vi "1 to 3 Down_movement_v11.vi"(1 "Input pixmap":u8[][](array[numeric]), 2 "start Column":i32) -> (3 "Total point":i32, 4 "moveLog(Row, Col.)":i32[][](array[numeric]), 5 "To:finish Col.":i32, 6 "TapN":dbl)   [LabVIEW 2016]
panel:
  out "i":i32
  out "1forward":u8[](array[numeric])
  out "2forward":u8[](array[numeric])
  out "RupPoint":dbl[](array[numeric]) format="%_3f"
  out "pointLog":u8[](array[numeric])
  out "min. root p.":u8
  out "3×3 point array":u8[][][](array[numeric])
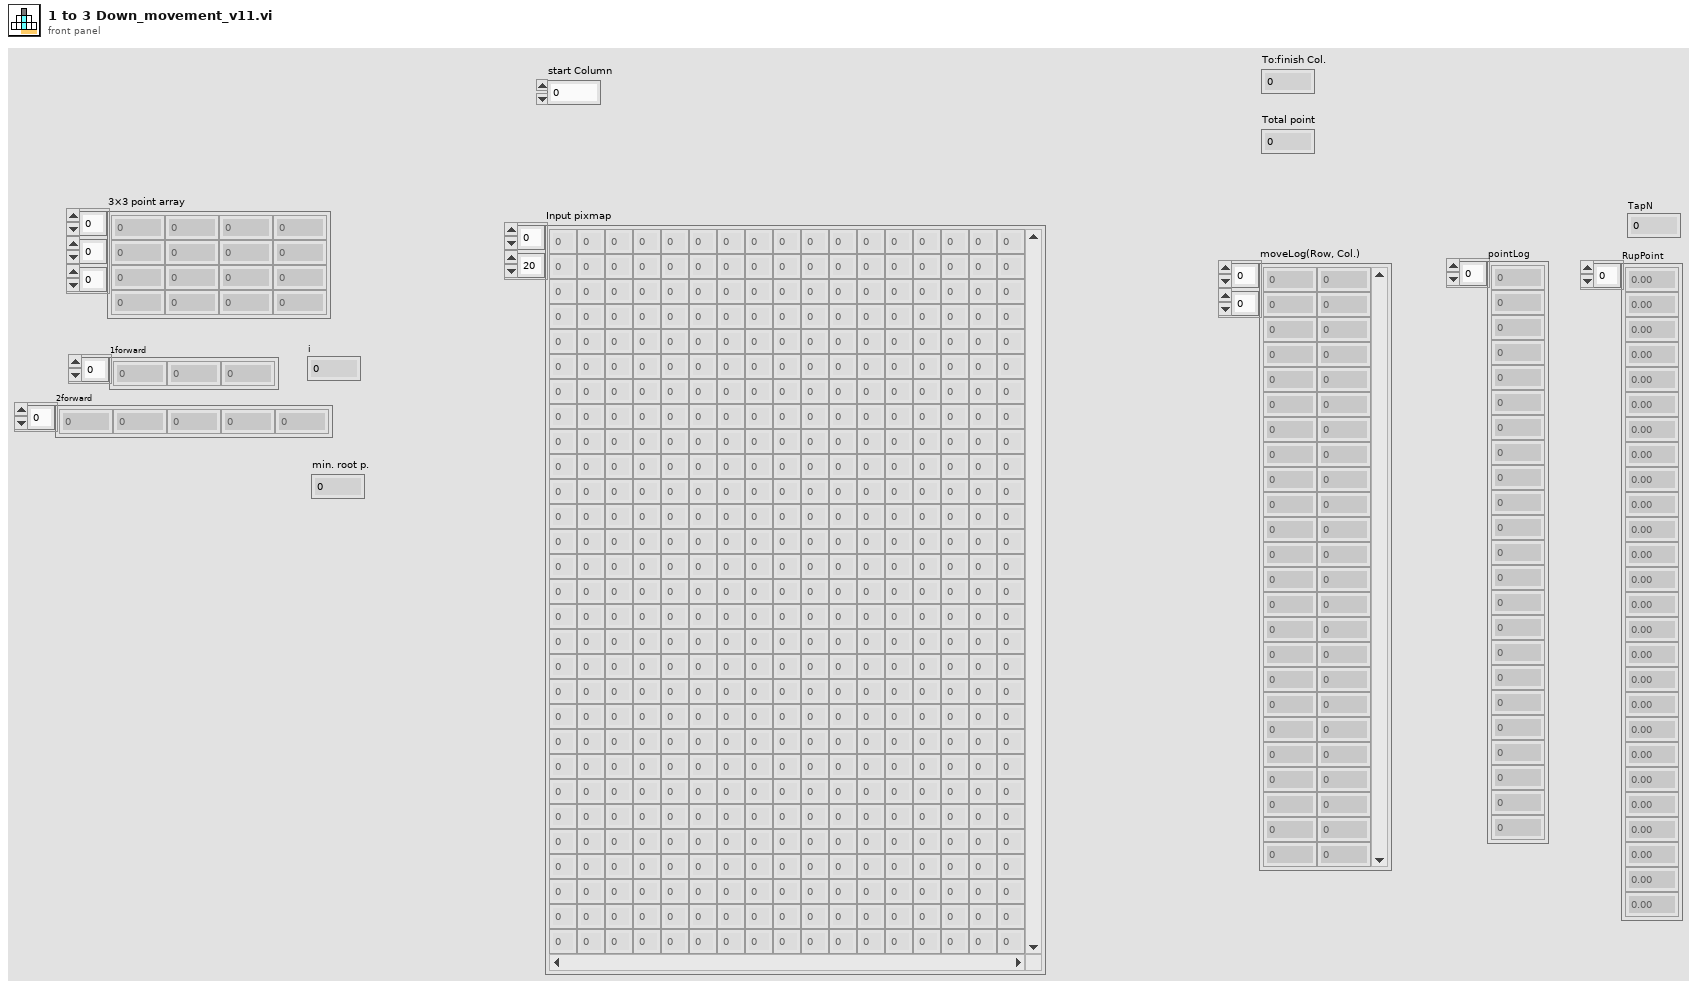
[diagram p1: front panel]
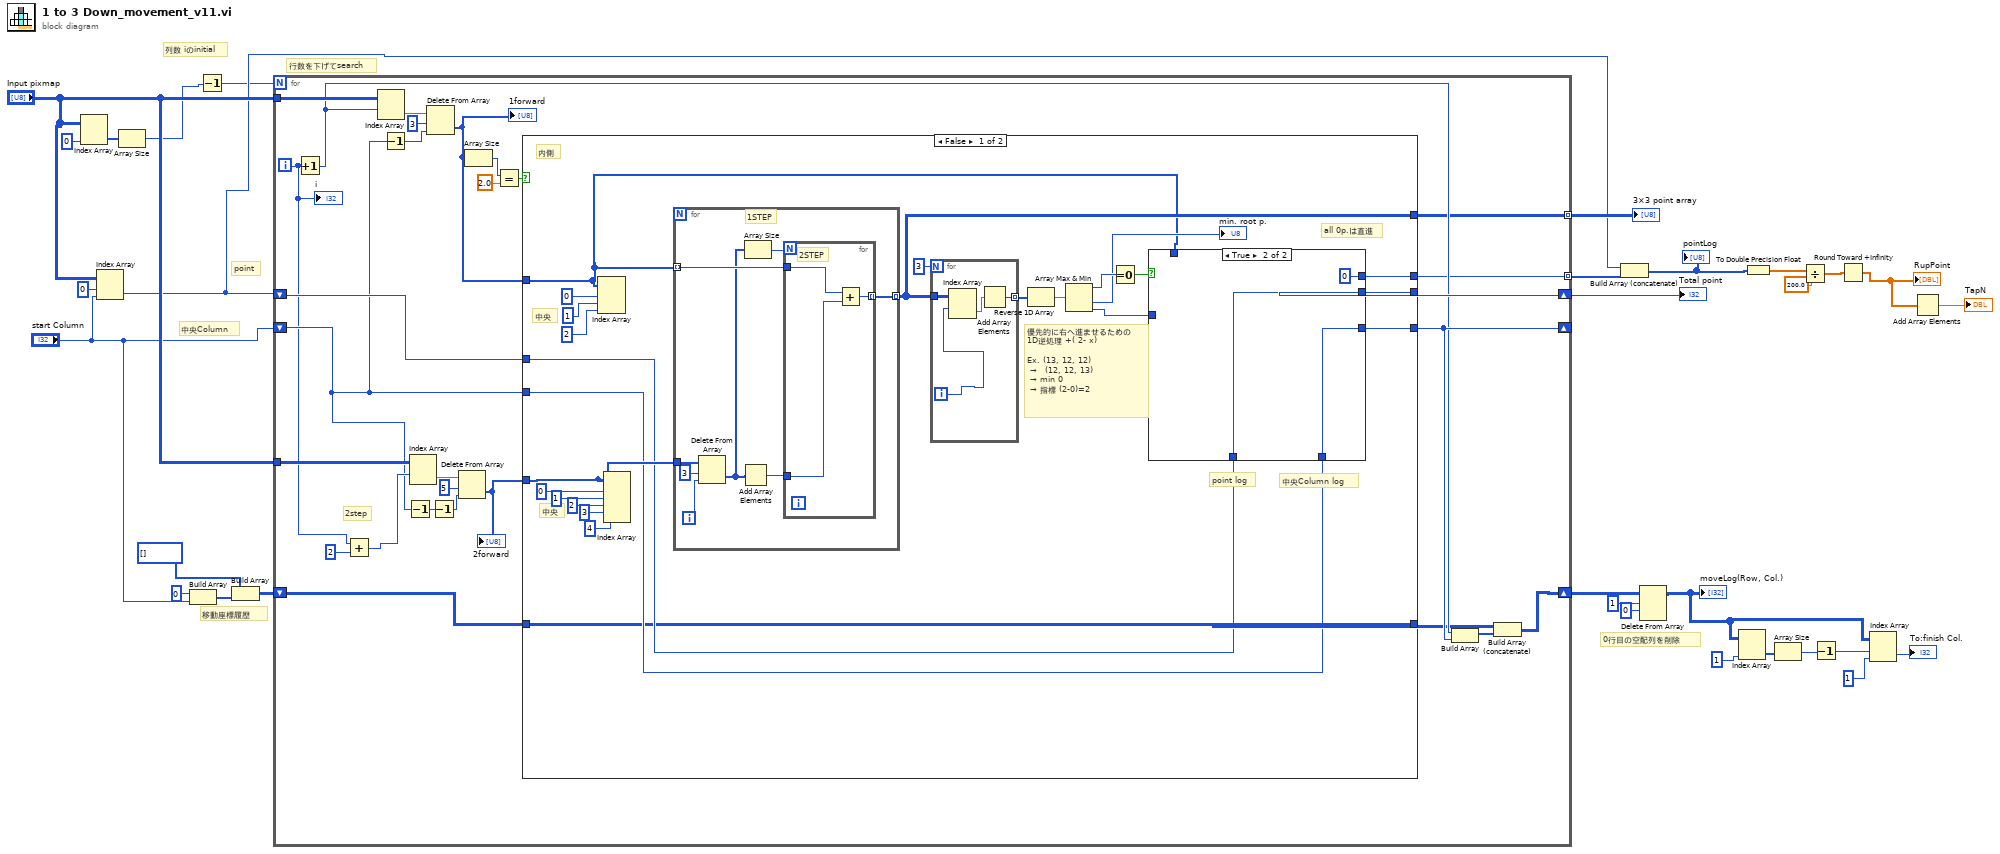
[diagram p0: block diagram]
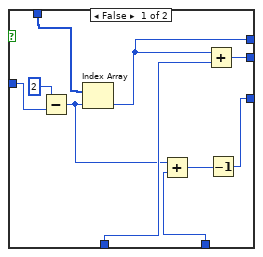
[diagram p2: hidden frame]
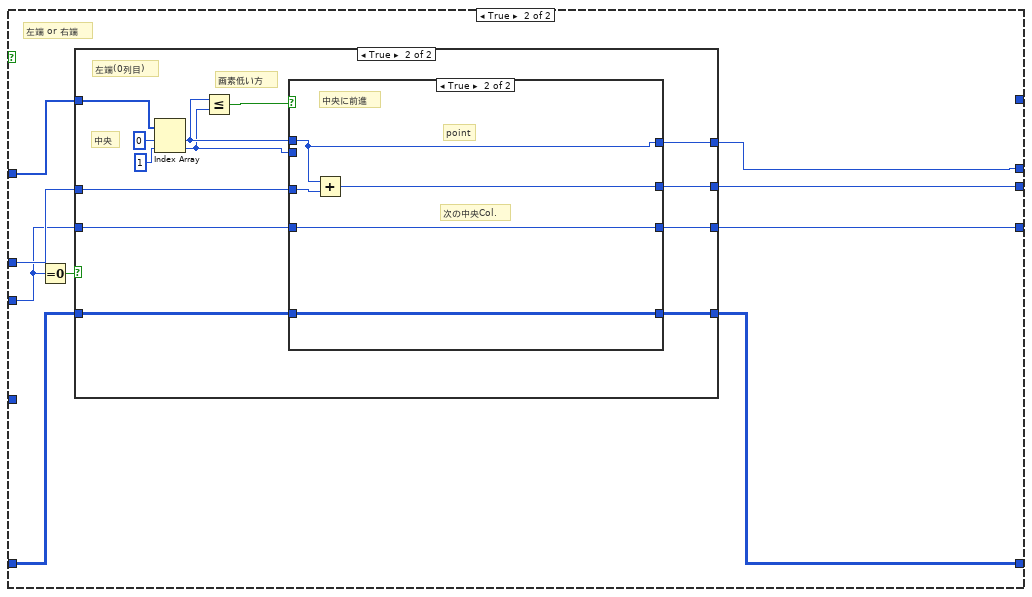
[diagram p3: hidden frame]
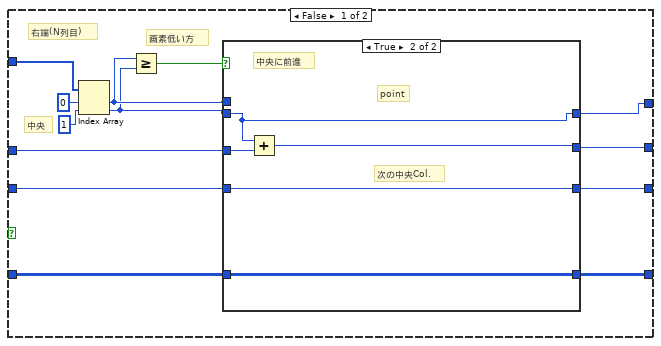
[diagram p4: hidden frame]
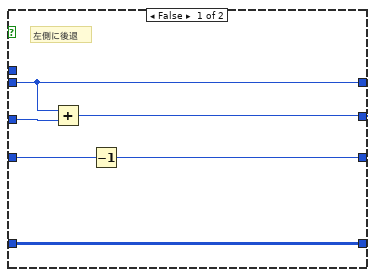
[diagram p5: hidden frame]
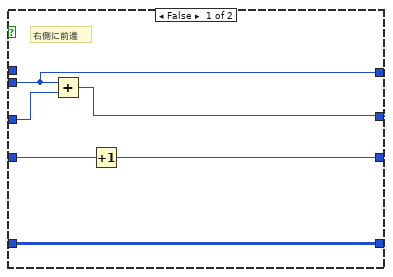
[diagram p6: hidden frame]
diagram:
  # "0行目の空配列を削除"
  # "移動座標履歴"
  # "中央Column"
  # "point"
  # "行数を下げてsearch"
  # "列数 iのinitial"
  n1 = Index Array(array="Input pixmap", index (col)=0 ("無効な指標 （列）")) -> (element=w29:u8[])  [unwired: 1 in]
  n2 = Index Array(array="Input pixmap", index (row)=0 ("指標 （行）"), index (col)="start Column") -> (element=w10:u8)
  n3 = Array Size(array=w29) -> (size(s)=w2:i32)
  n4 = Build Array(0 ("要素"), "start Column") -> (w27:i32[])
  n5 = Decrement(x=w2) -> (x-1=w1:i32)
  n6 = Build Array(i32[] [] ("要素"), w27) -> (w28:i32[][])
  n7 = for {
    N: w1 -> [_]
    tunnel: "Input pixmap" -> [w59]
    shift-right: [w51] -> w31
    shift-left: w10 -> [w52]
    shift-right: [w50] -> _
    shift-left: "start Column" -> [w38]
    shift-right: [w48] -> w25
    shift-left: w28 -> [w49]
    tunnel: "Input pixmap" -> [w40]
    tunnel: [w34] -> w14 mode=indexing
    tunnel: [w33] -> w9 mode=indexing
    i -> [w35]
    # "2step"
    n8 = Increment(x=w35) -> (x+1=w47:i32)
    n9 = Add(x=w35, y=2) -> (x+y=w39:i32)
    n10 = Index Array(array=w59, index (row)=w47) -> (element=w58:u8[])  [unwired: 1 in]
    n11 = Decrement(x=w38) -> (x-1=w56:i32)
    n12 = Decrement(x=w38) -> (x-1=w41:i32)
    n13 = Index Array(array=w40, index (row)=w39) -> (element=w37:u8[])  [unwired: 1 in]
    n14 = Delete From Array(array=w58, length=3 ("長さ"), index=w56) -> (deleted portion=w32:u8[])  [unwired: 1 out]
    "1forward" <- w32
    n15 = Decrement(x=w41) -> (x-1=w42:i32)
    n16 = Delete From Array(array=w37, length=5 ("長さ"), index=w42) -> (deleted portion=w36:u8[])  [unwired: 1 out]
    "2forward" <- w36
    n17 = Array Size(array=w32) -> (size(s)=w53:i32)
    n18 = Equal?(x=w53, y=2.0) -> (x = y?=w54:bool)
    n19 = case shown="False" w54 {
      tunnel: w32 -> [w61 w120]
      tunnel: w52 -> [w70 w119]
      tunnel: [w67 w118] -> w51
      tunnel: w38 -> [w69 w115]
      tunnel: [w66 w117] -> w50
      tunnel: [w68 w114] -> w45
      tunnel: w49 -> [w68 w113]
      tunnel: w36 -> [w75 _]
      tunnel: [w65 _] -> w34
      tunnel: [w60 w112] -> w33
      frame False {
        # "優先的に右へ進ませるための\n1D逆処理 +( 2- x)\n\nEx. (13, 12, 12)\n →　(12, 12, 13)\n → min 0\n → 指標 (2-0)=2"
        # "中央Column log"
        # "point log"
        # "all 0p.は直進"
        # "中央"
        # "中央"
        # "内側"
        n20 = Index Array(array=w61, index #1=0 ("指標"), index #2=1 ("指標"), index #3=2 ("指標")) -> ()  [unwired: 3 out]
        n21 = Index Array(array=w75, index #1=0 ("指標"), index #2=1 ("指標"), index #3=2 ("指標"), index #4=3 ("指標"), index #5=4 ("指標")) -> ()  [unwired: 5 out]
        n22 = for {
          tunnel: w61 -> [w108] mode=indexing
          tunnel: w75 -> [w106]
          tunnel: [w107] -> w65 mode=indexing
          i -> [w104]
          # "1STEP"
          n23 = Delete From Array(array=w106, length=3 ("長さ"), index=w104) -> (deleted portion=w101:u8[])  [unwired: 1 out]
          n24 = Add Array Elements(numeric array=w101) -> (sum=w102:u8)
          n25 = Array Size(array=w101) -> (size(s)=w103:i32)
          n26 = for {
            N: w103 -> [_]
            tunnel: w108 -> [w111]
            tunnel: [w110] -> w107 mode=indexing
            tunnel: w102 -> [w109]
            # "2STEP"
            n27 = Add(x=w111, y=w109) -> (x+y=w110:u8)
          }
        }
        n28 = for {
          N: 3 -> [_]
          tunnel: w65 -> [w86]
          tunnel: [w87] -> w63 mode=indexing
          i -> [w84]
          n29 = Index Array(array=w86, index (row)=w84) -> (element=w85:u8[])  [unwired: 1 in]
          n30 = Add Array Elements(numeric array=w85) -> (sum=w87:u8)
        }
        n31 = Reverse 1D Array(array=w63) -> (reversed array=w62:u8[])
        n32 = Array Max & Min(array=w62) -> (max value=w73:u8, min value=→"min. root p.":u8, min index (indices)=w74:i32)  [unwired: 1 out]
        n33 = Equal To 0?(x=w73) -> (x = 0?=w72:bool)
        n34 = case shown="True" w72 {
          tunnel: w70 -> [w97 w100]
          tunnel: w74 -> [w91 _]
          tunnel: w69 -> [w95 w99]
          tunnel: [w94 w100] -> w67
          tunnel: [w93 w99] -> w66
          tunnel: w61 -> [w90 _]
          tunnel: [w88 u8 0] -> w60
          frame False {
            n35 = Subtract(x=2, y=w91) -> (x-y=w89:i32)
            n36 = Index Array(array=w90, index=w89) -> (element=w88:u8)
            n37 = Add(x=w89, y=w95) -> (x+y=w96:i32)
            n38 = Add(x=w88, y=w97) -> (x+y=w94:u8)
            n39 = Decrement(x=w96) -> (x-1=w93:i32)
          }
          frame True {
          }
        }
      }
      frame True {
        # "左端 or 右端"
        n40 = Equal To 0?(x=w115) -> (x = 0?=w116:bool)
        n41 = case shown="True" w116 {
          tunnel: w120 -> [w131 w157]
          tunnel: w119 -> [w127 w154]
          tunnel: [w124 w153] -> w118
          tunnel: w115 -> [w126 w152]
          tunnel: [w123 w151] -> w117
          tunnel: [w122 w147] -> w114
          tunnel: w113 -> [w125 w146]
          tunnel: [w121 w145] -> w112
          frame False {
            # "中央"
            # "画素低い方"
            # "右端(N列目)"
            n42 = Index Array(array=w131, index #1=0 ("指標"), index #2=1 ("指標")) -> (element #1=w129:u8, element #2=w128:u8)
            n43 = Greater Or Equal?(x=w129, y=w128) -> (x >= y?=w130:bool)
            n44 = case shown="True" w130 {
              tunnel: w129 -> [_ _]
              tunnel: w127 -> [w135 w144]
              tunnel: [w139 w143] -> w124
              tunnel: w126 -> [w138 w142]
              tunnel: [w137 w142] -> w123
              tunnel: w128 -> [w134 w140]
              tunnel: [w136 w141] -> w122
              tunnel: w125 -> [w136 w141]
              tunnel: [w134 w140] -> w121
              frame False {
                # "左側に後退"
                n45 = Add(x=w134, y=w135) -> (x+y=w139:u8)
                n46 = Decrement(x=w138) -> (x-1=w137:i32)
              }
              frame True {
                # "中央に前進"
                # "次の中央Col."
                # "point"
                n47 = Add(x=w140, y=w144) -> (x+y=w143:u8)
              }
            }
          }
          frame True {
            # "中央"
            # "画素低い方"
            # "左端(0列目)"
            n48 = Index Array(array=w157, index #1=0 ("指標"), index #2=1 ("指標")) -> (element #1=w149:u8, element #2=w148:u8)
            n49 = Less Or Equal?(x=w149, y=w148) -> (x <= y?=w150:bool)
            n50 = case shown="True" w150 {
              tunnel: w149 -> [_ w164]
              tunnel: w154 -> [w163 w168]
              tunnel: [w162 w167] -> w153
              tunnel: w152 -> [w161 w166]
              tunnel: [w160 w166] -> w151
              tunnel: w148 -> [w158 _]
              tunnel: [w159 w165] -> w147
              tunnel: w146 -> [w159 w165]
              tunnel: [w158 w164] -> w145
              frame False {
                # "右側に前進"
                n51 = Add(x=w158, y=w163) -> (x+y=w162:u8)
                n52 = Increment(x=w161) -> (x+1=w160:i32)
              }
              frame True {
                # "中央に前進"
                # "次の中央Col."
                # "point"
                n53 = Add(x=w164, y=w168) -> (x+y=w167:u8)
              }
            }
          }
        }
      }
    }
    n54 = Build Array(w47, w50) -> (w46:i32[])
    n55 = Build Array (concatenate)(w45, w46) -> (w48:i32[][])
    "i" <- w35
  }
  "Total point" <- w31
  "3×3 point array" <- w14
  n56 = Build Array (concatenate)(w10, w9) -> (w5:u8[])
  "pointLog" <- w5
  n57 = Delete From Array(array=w25, length=1 ("長さ"), index (row)=0 ("指標 （行）")) -> (array with subset deleted=w19:i32[][])  [unwired: 1 in, 1 out]
  "moveLog(Row, Col.)" <- w19
  n58 = Index Array(array=w19, index (col)=1 ("指標 （行）")) -> (element=w23:i32[])  [unwired: 1 in]
  n59 = To Double Precision Float(number=w5) -> (double precision float=w8:dbl[])
  n60 = Array Size(array=w23) -> (size(s)=w16:i32)
  n61 = Divide(x=w8, y=200.0) -> (x/y=w6:dbl[])
  n62 = Decrement(x=w16) -> (x-1=w15:i32)
  n63 = Round Toward +Infinity(x=w6) -> (ceil(x): smallest int >= x=w4:dbl[])
  "RupPoint" <- w4
  n64 = Index Array(array=w19, index (row)=w15, index (col)=1 ("指標 （行）")) -> (element=→"To:finish Col.":i32)
  n65 = Add Array Elements(numeric array=w4) -> (sum=→"TapN":dbl)
